vi "Update_Item.vi"(8 "error in (no error)":errorcluster, 11 "IB_Tree_Item_Proj in":refnum<class "IB_Tree_Item_Proj.lvclass">) -> (0 "error out":errorcluster, 3 "IB_Tree_Item_Proj out":refnum<class "IB_Tree_Item_Proj.lvclass">)   [LabVIEW 2020, in "IB_Tree_Item_Proj.lvclass"]
uses:
  <vilib>/AppBuilder/IB_Classes/Tree_Item_Proj/IB_Tree_Item_Proj.lvclass
  <vilib>/AppBuilder/IB_Classes/Tree_Item_Proj/IB_Tree_Item_Proj.lvclass/IB_Tree_Item_Proj.ctl
  <vilib>/AppBuilder/IB_Classes/Tree_Item/IB_Tree_Item.lvclass
  e:/builds/penguin/labview/branches/2020/dev/dist/vi.lib/AppBuilder/IB_Classes/Tree_Item/IB_Tree_Item.lvclass
  e:/builds/penguin/labview/branches/2020/dev/dist/vi.lib/AppBuilder/IB_Classes/Tree_Item_Proj/IB_Tree_Item_Proj.lvclass
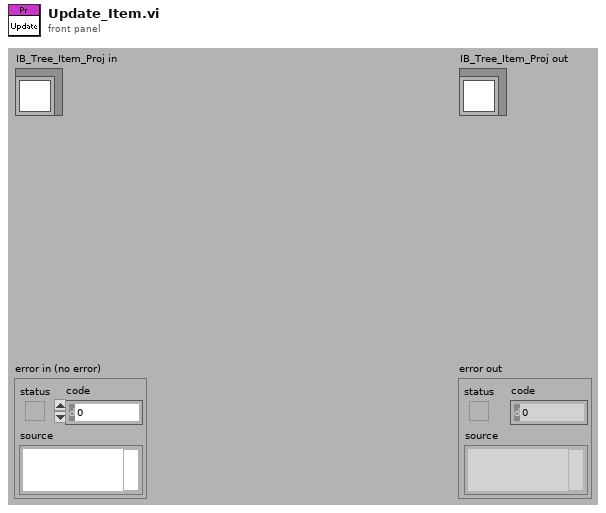
[diagram p1: front panel]
types:
  T1 = typedef "IB_Tree_Item.ctl" = cluster{"symbol index":i32, "child tag":string, "parentTag":string, "left cell name":string}
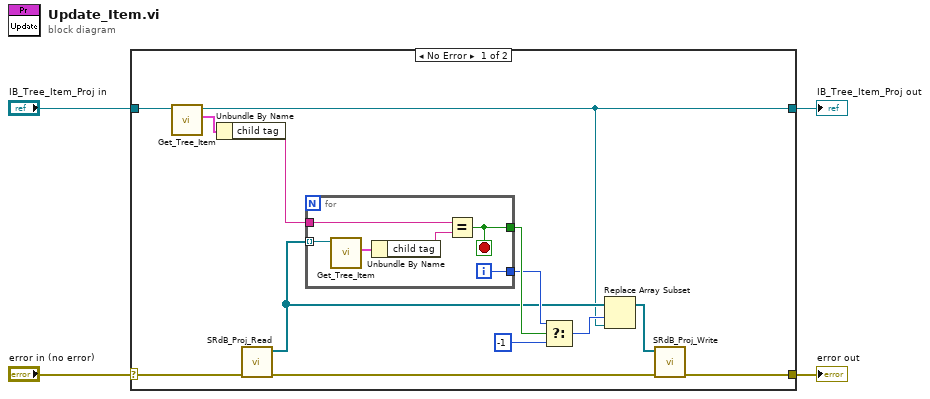
[diagram p0: block diagram]
diagram:
  n1 = case shown="No Error" "error in (no error)" {
    selector: "error in (no error)" -> [w8 w25]
    tunnel: [w7 w25] -> w3
    tunnel: [w5 w24] -> w1
    tunnel: "IB_Tree_Item_Proj in" -> [w6 w24]
    frame No Error {
      n2 = call <vilib>:"Get_Tree_Item.vi"("IB_TreeItem in"=w6) -> ("data"=w14:T1, "IB_TreeItem out"=w5:refnum<class "IB_Tree_Item_Proj.lvclass">)  [unwired: 8 in, 1 out]
      n3 = Unbundle By Name(w14) -> ("child tag"=w13:string)
      n4 = call <resource>:"SRdB_Proj_Read.vi"("error in (no error)"=w8) -> ("error out"=w9:errorcluster, "Proj Items"=w12:refnum<class "IB_Tree_Item_Proj.lvclass">[])  [unwired: 9 in]
      n5 = for {
        tunnel: w12 -> [w19] mode=indexing
        tunnel: w13 -> [w22]
        tunnel: [w21] -> w17
        tunnel: [w20] -> w16
        i -> [w20]
        stop <- w21 stop-if-true
        n6 = call <vilib>:"Get_Tree_Item.vi"("IB_TreeItem in"=w19) -> ("data"=w18:T1)  [unwired: 8 in, 2 out]
        n7 = Unbundle By Name(w18) -> ("child tag"=w23:string)
        n8 = Equal?(x=w22, y=w23) -> (x = y?=w21:bool)
      }
      n9 = Select(t=w16, s=w17, f=-1) -> (s? t:f=w10:i32)
      n10 = Replace Array Subset(array=w12, new element=w5, index=w10) -> (w11:refnum<class "IB_Tree_Item_Proj.lvclass">[])
      n11 = call <resource>:"SRdB_Proj_Write.vi"("error in (no error)"=w9, "Proj Items"=w11) -> ("error out"=w7:errorcluster)  [unwired: 9 in]
    }
    frame Error {
    }
  }
  "error out" <- w3
  "IB_Tree_Item_Proj out" <- w1
